vi "NameMap-Check.vi"(8 "error in (no error)":errorcluster, 10 "Name":string, 11 "NameMap in":T1) -> (0 "error out":errorcluster, 2 "OriginName":string, 3 "NameMap out":T1)   [LabVIEW 2019, in "lv-apt-json-file.lvlib"]
uses:
  lv-apt-json-file.lvlib
  Typedef/Def-NameMap.ctl
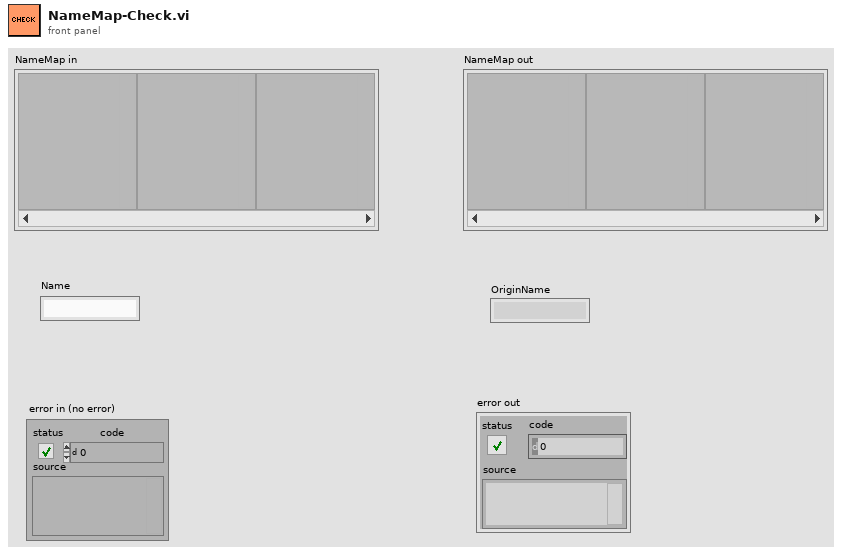
[diagram p1: front panel]
types:
  T1 = typedef "lv-apt-json-file.lvlib/Def-NameMap.ctl" = variant[]
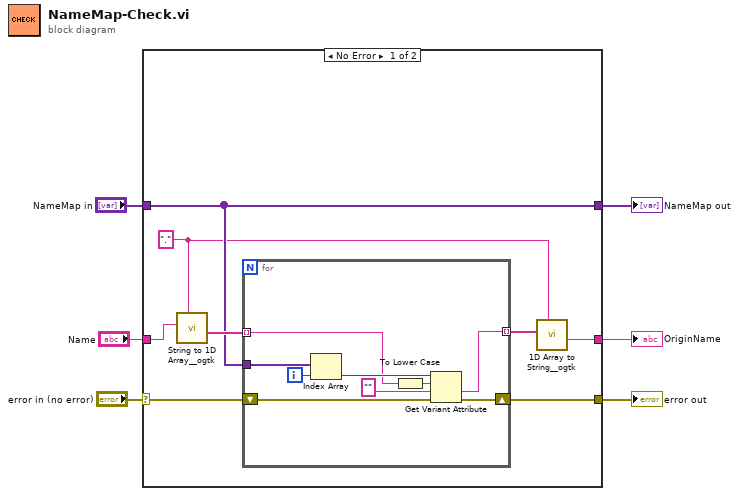
[diagram p0: block diagram]
diagram:
  n1 = case shown="No Error" "error in (no error)" {
    selector: "error in (no error)" -> [w13 w26]
    tunnel: "Name" -> [w14 w24]
    tunnel: [w10 w25] -> w5
    tunnel: [w12 w26] -> w3
    tunnel: "NameMap in" -> [w10 w25]
    tunnel: [w7 w24] -> w1
    frame No Error {
      w8 = "." ("delimiter (Tab)")
      n2 = call <userlib>:"String to 1D Array__ogtk.vi"("delimiter (Tab)"=w8, "string"=w14) -> ("Array of Strings"=w11:string[])  [unwired: 9 in]
      n3 = for {
        tunnel: w11 -> [w20] mode=indexing
        shift-right: [w19] -> w12
        shift-left: w13 -> [w18]
        tunnel: w10 -> [w16]
        tunnel: [w15] -> w9 mode=indexing
        i -> [w23]
        n4 = Index Array(array=w16, index=w23) -> (element=w22:variant)
        n5 = To Lower Case(string=w20) -> (all lower case string=w17:string)
        n6 = Get Variant Attribute(Variant=w22, name=w17, default value (empty Variant)="" ("delimiter (Tab)"), error in=w18) -> (value=w15:string, error out=w19:errorcluster)  [unwired: 2 out]
      }
      n7 = call <userlib>:"1D Array to String__ogtk.vi"("delimiter (Tab)"=w8, "Array of Strings"=w9) -> ("delimited string"=w7:string)  [unwired: 9 in]
    }
    frame Error {
    }
  }
  "NameMap out" <- w5
  "error out" <- w3
  "OriginName" <- w1
